vi "Begin.vi"(8 "error in":errorcluster) -> (0 "error out":errorcluster)   [LabVIEW 2018]
doc: "Called before other user functions, this VI is expected to open initial I/O refnums, load in file data, and do all program initialization. Notice that the <B>error out</B> terminal is simply used for data flow. Wiring it to other structures or subVIs ensures that this VI runs first."
uses:
  <vilib>/Rock Robotics/WPI/DriverStation/WPI_DriverStationRobotMode2.ctl
  <vilib>/Rock Robotics/WPI/Joystick/WPI_JoystickDeviceEnum.ctl
  <vilib>/Rock Robotics/WPI/Solenoid/WPI_SolenoidChannel.ctl
  Robot Global Data.vi
  <vilib>/Rock Robotics/WPI/Solenoid/WPI_SolenoidOpenSingle.vi
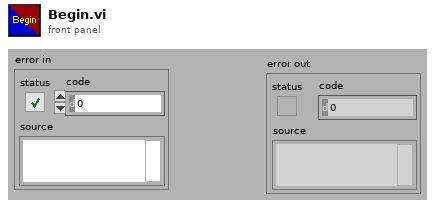
[diagram p1: front panel]
types:
  T1 = typedef "WPI_SolenoidChannel.ctl" = enum8{"Solenoid 0", "Solenoid 1", "Solenoid 2", "Solenoid 3", "Solenoid 4", "Solenoid 5", "Solenoid 6", "Solenoid 7", "Invalid"}
  T2 = typedef "WPI_JoystickDeviceEnum.ctl" = enum16{"USB 0", "USB 1", "USB 2", "USB 3", "USB 4", "USB 5"}
  T3 = typedef "WPI_DriverStationRobotMode2.ctl" = enum16{"Autonomous Disabled", "Autonomous Enabled", "Teleop Disabled", "Teleop Enabled", "Disconnected", "Finish", "Test Disabled", "Test Enabled", "Emergency Stopped"}
  T4 = typedef "WPI_MotorControlDeviceRef.ctl" = cluster{"DeviceStatus":errorcluster, "Type":T5, "PWM":cluster{"PWM Channel":T6, "DeadBand":T7}, "CAN":cluster{"Device Number":u8, "SetOutput VI Ref":variant, "GetOutput VI Ref":variant, "Enable VI Ref":variant, "Disable VI Ref":variant, "Data":variant}, "Invert":bool, "DIO PWM":cluster{"PWM \"Enable\" Channel":T6, "DIOChannel":T8, "PWM Rate":dbl}}
  T5 = typedef "WPI_MotorControlType.ctl" = enum16{"PWM", "CAN", "DIO PWM"}
  T6 = typedef "FPGA_DIOPWMChannel.ctl" = enum8{"PWM 0", "PWM 1", "PWM 2", "PWM 3", "PWM 4", "PWM 5", "PWM 6", "PWM 7", "PWM 8", "PWM 9", "PWM MXP 0", "PWM MXP 1", "PWM MXP 2", "PWM MXP 3", "PWM MXP 4", "PWM MXP 5", "PWM MXP 6", "PWM MXP 7", "PWM MXP 8", "PWM MXP 9", "Invalid"}
  T7 = typedef "WPI_PWMDeadband.ctl" = cluster{"Name":string, "maxPositivePwm":i32, "minPositivePwm":i32, "centerPwm":i32, "maxNegativePwm":i32, "minNegativePwm":i32, "angularRange":u16}
  T8 = typedef "FPGA_DIOChannel.ctl" = enum8{"DIO 0", "DIO 1", "DIO 2", "DIO 3", "DIO 4", "DIO 5", "DIO 6", "DIO 7", "DIO 8", "DIO 9", "DIO MXP 0", "DIO MXP 1", "DIO MXP 2", "DIO MXP 3", "DIO MXP 4", "DIO MXP 5", "DIO MXP 6", "DIO MXP 7", "DIO MXP 8", "DIO MXP 9", "DIO MXP 10", "DIO MXP 11", "DIO MXP 12", "DIO MXP 13", "DIO MXP 14", "DIO MXP 15", "SPI Port CS1", "SPI Port CS2", "SPI Port CS3", "SPI Port MISO", "SPI Port MOSI", "Invalid"}
  T9 = typedef "WPI_JoystickDevRef.ctl" = cluster{"Device":T2}
  T10 = typedef "WPI_SolenoidDevRef.ctl" = cluster{"DevStatus":errorcluster, "Pneumatics Control Module":u8, "Forward Solenoid Channel":T1, "Reverse Solenoid Channel":T1}
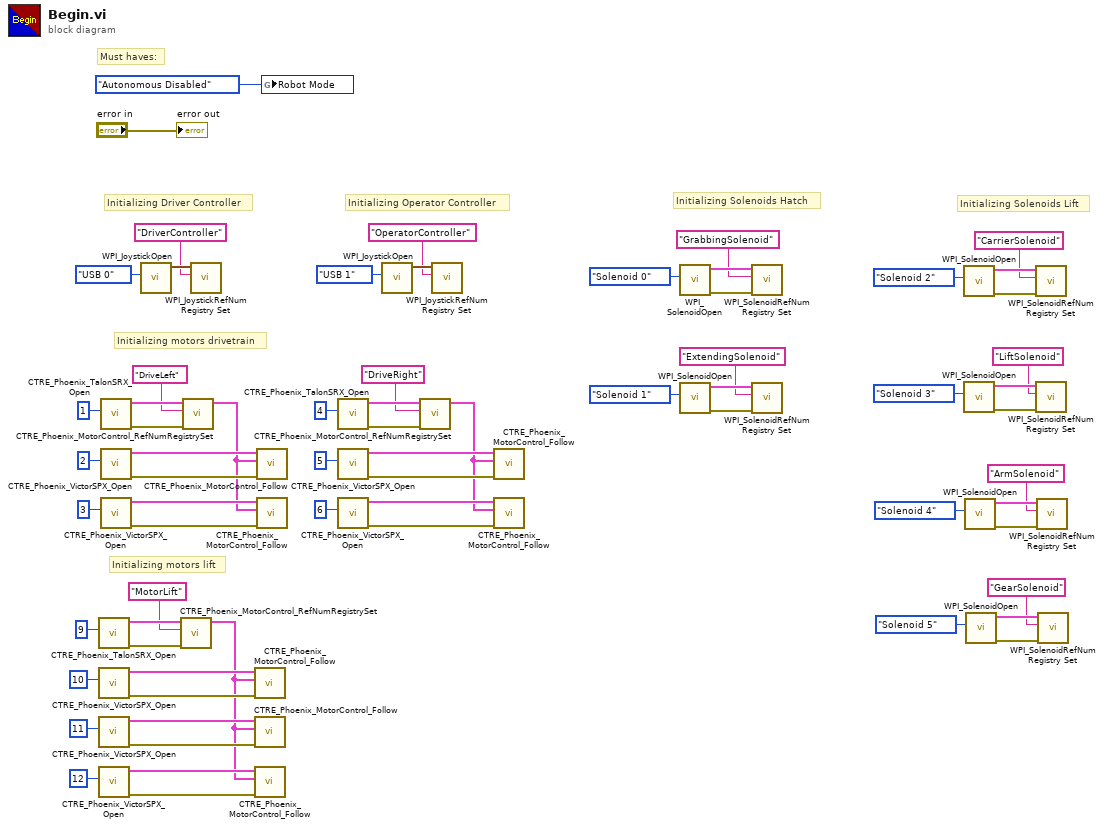
[diagram p0: block diagram]
diagram:
  # "Initializing motors lift"
  # "Initializing Solenoids Lift"
  # "Initializing Solenoids Hatch"
  # "Initializing Operator Controller"
  # "Initializing Driver Controller"
  # "Initializing motors drivetrain"
  # "Must haves:"
  n1 = call <vilib>:"CTRE_Phoenix_TalonSRX_Open.vi"("Device Number"=u8 9) -> ("error out"=w7:errorcluster, "CAN Talon SRX Ref"=w6:T4)  [unwired: 9 in]
  n2 = call <vilib>:"CTRE_Phoenix_VictorSPX_Open.vi"("Device Number"=u8 10) -> ("error out"=w11:errorcluster, "CAN Talon SRX Ref"=w10:T4)  [unwired: 9 in]
  n3 = call <vilib>:"CTRE_Phoenix_VictorSPX_Open.vi"("Device Number"=u8 11) -> ("error out"=w9:errorcluster, "CAN Talon SRX Ref"=w8:T4)  [unwired: 9 in]
  n4 = call <vilib>:"CTRE_Phoenix_VictorSPX_Open.vi"("Device Number"=u8 12) -> ("error out"=w3:errorcluster, "CAN Talon SRX Ref"=w2:T4)  [unwired: 9 in]
  n5 = call <vilib>:"CTRE_Phoenix_TalonSRX_Open.vi"("Device Number"=u8 1) -> ("error out"=w59:errorcluster, "CAN Talon SRX Ref"=w58:T4)  [unwired: 9 in]
  n6 = call <vilib>:"CTRE_Phoenix_VictorSPX_Open.vi"("Device Number"=u8 2) -> ("error out"=w63:errorcluster, "CAN Talon SRX Ref"=w62:T4)  [unwired: 9 in]
  n7 = call <vilib>:"CTRE_Phoenix_VictorSPX_Open.vi"("Device Number"=u8 3) -> ("error out"=w61:errorcluster, "CAN Talon SRX Ref"=w60:T4)  [unwired: 9 in]
  n8 = call <vilib>:"WPI_JoystickOpen.vi"("JoystickDevice"=WPI_JoystickDeviceEnum."USB 0") -> ("JoystickDevRef"=w42:T9)  [unwired: 10 in]
  n9 = call <vilib>:"CTRE_Phoenix_MotorControl_RefNumRegistrySet.vi"("error in (no error)"=w7, "refnum name"="MotorLift", "PhoenixMotorControlDevRef"=w6) -> ("PhoenixMotorControlDevRef"=w1:T4)  [unwired: 7 in, 1 out]
  n10 = call <vilib>:"CTRE_Phoenix_MotorControl_RefNumRegistrySet.vi"("error in (no error)"=w59, "refnum name"="DriveLeft", "PhoenixMotorControlDevRef"=w58) -> ("PhoenixMotorControlDevRef"=w56:T4)  [unwired: 7 in, 1 out]
  n11 = call <vilib>:"WPI_JoystickRefNum Registry Set.vi"("refnum name"="DriverController", "JoystickDevRef"=w42) -> ()  [unwired: 8 in, 2 out]
  n12 = call <vilib>:"CTRE_Phoenix_MotorControl_Follow.vi"("error in (no error)"=w11, "Master Controller to Follow"=w1, "PhoenixMotorControlDevRef"=w10) -> ()  [unwired: 7 in, 2 out]
  n13 = call <vilib>:"CTRE_Phoenix_MotorControl_Follow.vi"("error in (no error)"=w9, "Master Controller to Follow"=w1, "PhoenixMotorControlDevRef"=w8) -> ()  [unwired: 7 in, 2 out]
  n14 = call <vilib>:"CTRE_Phoenix_MotorControl_Follow.vi"("error in (no error)"=w3, "Master Controller to Follow"=w1, "PhoenixMotorControlDevRef"=w2) -> ()  [unwired: 7 in, 2 out]
  n15 = call <vilib>:"CTRE_Phoenix_MotorControl_Follow.vi"("error in (no error)"=w63, "Master Controller to Follow"=w56, "PhoenixMotorControlDevRef"=w62) -> ()  [unwired: 7 in, 2 out]
  n16 = call <vilib>:"CTRE_Phoenix_MotorControl_Follow.vi"("error in (no error)"=w61, "Master Controller to Follow"=w56, "PhoenixMotorControlDevRef"=w60) -> ()  [unwired: 7 in, 2 out]
  n17 = global write "Robot Global Data.vi" "Robot Mode"(WPI_DriverStationRobotMode2."Autonomous Disabled" ("Robot Mode")) -> ()
  n18 = call <vilib>:"CTRE_Phoenix_TalonSRX_Open.vi"("Device Number"=u8 4) -> ("error out"=w48:errorcluster, "CAN Talon SRX Ref"=w47:T4)  [unwired: 9 in]
  n19 = call <vilib>:"CTRE_Phoenix_VictorSPX_Open.vi"("Device Number"=u8 5) -> ("error out"=w52:errorcluster, "CAN Talon SRX Ref"=w51:T4)  [unwired: 9 in]
  n20 = call <vilib>:"CTRE_Phoenix_VictorSPX_Open.vi"("Device Number"=u8 6) -> ("error out"=w50:errorcluster, "CAN Talon SRX Ref"=w49:T4)  [unwired: 9 in]
  n21 = call <vilib>:"WPI_JoystickOpen.vi"("JoystickDevice"=WPI_JoystickDeviceEnum."USB 1") -> ("JoystickDevRef"=w41:T9)  [unwired: 10 in]
  n22 = call <vilib>:"CTRE_Phoenix_MotorControl_RefNumRegistrySet.vi"("error in (no error)"=w48, "refnum name"="DriveRight", "PhoenixMotorControlDevRef"=w47) -> ("PhoenixMotorControlDevRef"=w45:T4)  [unwired: 7 in, 1 out]
  n23 = call <vilib>:"WPI_JoystickRefNum Registry Set.vi"("refnum name"="OperatorController", "JoystickDevRef"=w41) -> ()  [unwired: 8 in, 2 out]
  n24 = call <vilib>:"CTRE_Phoenix_MotorControl_Follow.vi"("error in (no error)"=w52, "Master Controller to Follow"=w45, "PhoenixMotorControlDevRef"=w51) -> ()  [unwired: 7 in, 2 out]
  n25 = call <vilib>:"CTRE_Phoenix_MotorControl_Follow.vi"("error in (no error)"=w50, "Master Controller to Follow"=w45, "PhoenixMotorControlDevRef"=w49) -> ()  [unwired: 7 in, 2 out]
  n26 = call-poly <vilib>:"WPI_SolenoidOpen.vi"("Solenoid Channel"=WPI_SolenoidChannel."Solenoid 0") -> ("error out"=w38:errorcluster, "SolenoidDevRef"=w37:T10)  [unwired: 9 in]
  n27 = call-poly <vilib>:"WPI_SolenoidOpen.vi"("Solenoid Channel"=WPI_SolenoidChannel."Solenoid 1") -> ("error out"=w34:errorcluster, "SolenoidDevRef"=w33:T10)  [unwired: 9 in]
  n28 = call <vilib>:"WPI_SolenoidRefNum Registry Set.vi"("error in (no error)"=w38, "refnum name"="GrabbingSolenoid", "SolenoidDevRef"=w37) -> ()  [unwired: 7 in, 2 out]
  n29 = call <vilib>:"WPI_SolenoidRefNum Registry Set.vi"("error in (no error)"=w34, "refnum name"="ExtendingSolenoid", "SolenoidDevRef"=w33) -> ()  [unwired: 7 in, 2 out]
  n30 = call-poly <vilib>:"WPI_SolenoidOpen.vi"("Solenoid Channel"=WPI_SolenoidChannel."Solenoid 2") -> ("error out"=w30:errorcluster, "SolenoidDevRef"=w29:T10)  [unwired: 9 in]
  n31 = call-poly <vilib>:"WPI_SolenoidOpen.vi"("Solenoid Channel"=WPI_SolenoidChannel."Solenoid 3") -> ("error out"=w26:errorcluster, "SolenoidDevRef"=w25:T10)  [unwired: 9 in]
  n32 = call-poly <vilib>:"WPI_SolenoidOpen.vi"("Solenoid Channel"=WPI_SolenoidChannel."Solenoid 4") -> ("error out"=w22:errorcluster, "SolenoidDevRef"=w21:T10)  [unwired: 9 in]
  n33 = call-poly <vilib>:"WPI_SolenoidOpen.vi"("Solenoid Channel"=WPI_SolenoidChannel."Solenoid 5") -> ("error out"=w18:errorcluster, "SolenoidDevRef"=w17:T10)  [unwired: 9 in]
  n34 = call <vilib>:"WPI_SolenoidRefNum Registry Set.vi"("error in (no error)"=w30, "refnum name"="CarrierSolenoid", "SolenoidDevRef"=w29) -> ()  [unwired: 7 in, 2 out]
  n35 = call <vilib>:"WPI_SolenoidRefNum Registry Set.vi"("error in (no error)"=w26, "refnum name"="LiftSolenoid", "SolenoidDevRef"=w25) -> ()  [unwired: 7 in, 2 out]
  n36 = call <vilib>:"WPI_SolenoidRefNum Registry Set.vi"("error in (no error)"=w22, "refnum name"="ArmSolenoid", "SolenoidDevRef"=w21) -> ()  [unwired: 7 in, 2 out]
  n37 = call <vilib>:"WPI_SolenoidRefNum Registry Set.vi"("error in (no error)"=w18, "refnum name"="GearSolenoid", "SolenoidDevRef"=w17) -> ()  [unwired: 7 in, 2 out]
  "error out" <- "error in"
